vi "Get Config.vi"(8 "error in (no error)":errorcluster, 11 "Reference":refnum<vi>) -> (0 "error out":errorcluster, 1 "Is DataGrid?":bool, 3 "DataGrid Config":refnum<class "DataGrid Config.lvclass">)   [LabVIEW 2018, in "DataGrid Config.lvclass"]
uses:
  DataGrid Config.lvclass
  Data Type Classes/Generic/Generic Data Type.lvclass
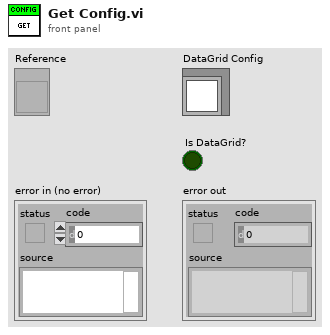
[diagram p1: front panel]
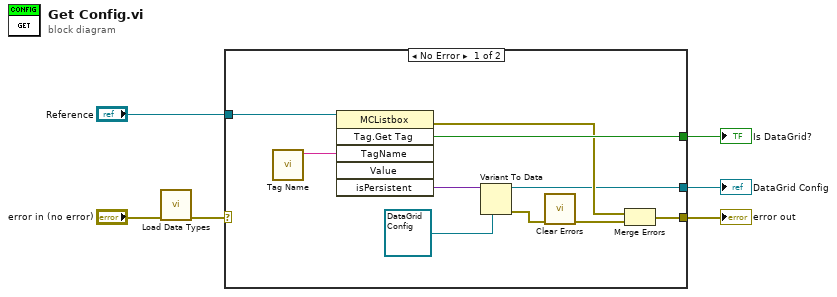
[diagram p0: block diagram]
diagram:
  n1 = call "Load Data Types.vi"("error in (no error)"="error in (no error)") -> ("error out"=w1:errorcluster)  [unwired: 8 in, 2 out]
  n2 = case shown="No Error" w1 {
    selector: w1 -> [_ w17]
    tunnel: [w9 w17] -> w6
    tunnel: [w15 _] -> w5
    tunnel: [w8 _] -> w4
    tunnel: "Reference" -> [w7 _]
    frame No Error {
      n3 = call "Tag Name.vi"() -> ("String"=w16:string)  [unwired: 11 in]
      n4 = invoke class="MCListbox" method="Tag.Get Tag"(reference=w7, "TagName"=w16) -> (error out=w11:errorcluster, "GetTag"=w15:bool, "isPersistent"=w14:variant)  [unwired: 4 in, 3 out]
      n5 = Variant To Data(type=refnum<class "DataGrid Config.lvclass"> refnum ("DataGrid Config"), Variant=w14) -> (data=w8:refnum<class "DataGrid Config.lvclass">, error out=w12:errorcluster)  [unwired: 1 in]
      n6 = call <vilib>:"Clear Errors.vi"("error in (no error)"=w12) -> ("error out"=w10:errorcluster)  [unwired: 5 in, 1 out]
      n7 = Merge Errors(w11, w10) -> (w9:errorcluster)
    }
    frame Error {
    }
  }
  "error out" <- w6
  "Is DataGrid?" <- w5
  "DataGrid Config" <- w4
